vi "Account holder name.vi"(11 "Module Data in":T1) -> (2 "Withdrawal Complete Message":string)   [LabVIEW 2016]
doc: "Index account holder first and last names and display them in the main menu message."
uses:
  Controls/UI Controls.ctl
  Controls/ATM Messages.ctl
  Controls/Transaction Status.ctl
  Controls/User Input Data.ctl
  Controls/Module Data.ctl
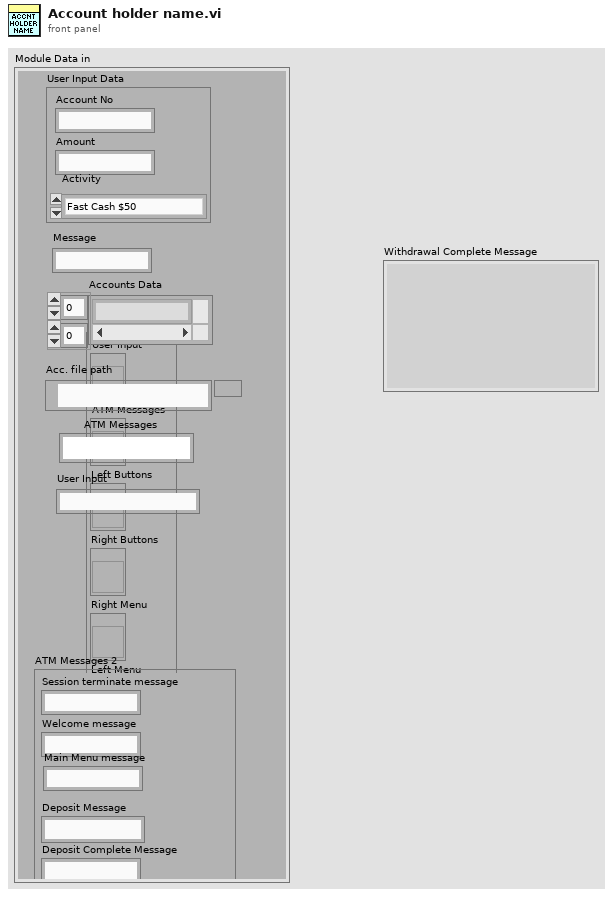
[diagram p1: front panel]
types:
  T1 = typedef "Module Data.ctl" = cluster{"UI Controls":T2, "ATM Messages 2":T3, "User Input":string, "ATM Messages":string, "Acc. file path":path, "Accounts Data":string[][], "User Input Data":T4, "Message":string}
  T2 = typedef "UI Controls.ctl" = cluster{"ATM Messages":refnum<vi>, "User Input":refnum<vi>, "Right Buttons":refnum<vi>, "Right Menu":refnum<vi>, "Left Buttons":refnum<vi>, "Left Menu":refnum<vi>, "Card Simulator":refnum<vi>, "Enter":refnum<vi>}
  T3 = typedef "ATM Messages.ctl" = cluster{"Session terminate message":string, "Welcome message":string, "Deposit Message":string, "Deposit Complete Message":string, "Withdrawal Message":string, "Withdrawal Complete Message":string, "Balance Inquiry Message":string, "Account verification failed message":string, "Withdrawal failed message":string, "Card Inserted":string, "Main Menu message":string}
  T4 = typedef "User Input Data.ctl" = cluster{"Account No":string, "Amount":string, "Activity":T5}
  T5 = typedef "Transaction Status.ctl" = enum16{"Fast Cash $50", "Withdrawal?", "Deposit?", "Account Number?"}
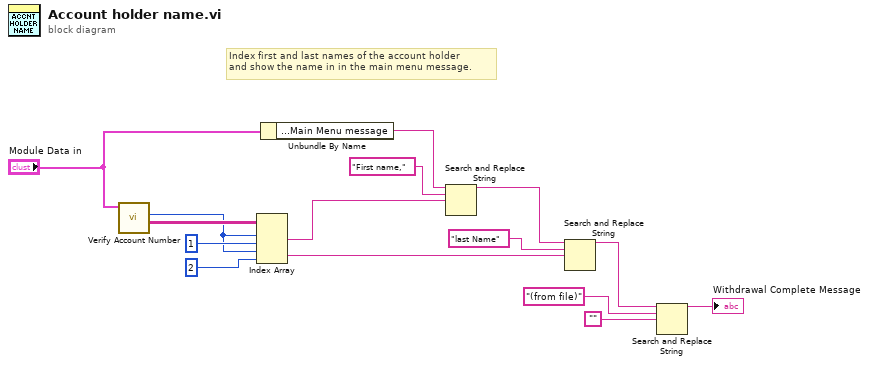
[diagram p0: block diagram]
diagram:
  # "Index first and last names of the account holder\nand show the name in in the main menu message."
  n1 = call "Verify Account Number.vi"("Module Data"="Module Data in") -> ("Accounts all data"=w13:string[][], "Index account no."=w11:i32)  [unwired: 6 in, 3 out]
  n2 = Index Array(array=w13, index (row) #1=w11, index (col) #1=1 ("disabled index (col)"), index (row) #2=w11, index (col) #2=2 ("disabled index (col)")) -> (element #1=w9:string, element #2=w7:string)
  n3 = Unbundle By Name("Module Data in") -> ("ATM Messages 2.Main Menu message"=w5:string)
  n4 = Search and Replace String(input string=w5, search string="First name," ("search string/char (-)"), replace string=w9) -> (result string=w3:string)  [unwired: 5 in, 3 out]
  n5 = Search and Replace String(input string=w3, search string="last Name" ("search string/char (-)"), replace string=w7) -> (result string=w2:string)  [unwired: 5 in, 3 out]
  n6 = Search and Replace String(input string=w2, search string="(from file)" ("search string/char (-)"), replace string="") -> (result string=→"Withdrawal Complete Message":string)  [unwired: 5 in, 3 out]
